vi "_Read RT Table.vi"(4 "error in (no error)":errorcluster, 6 "key":string, 7 "Simulator":bool) -> (0 "error out":errorcluster, 1 "Table":dbl[][](array[numeric]))   [LabVIEW 2015]
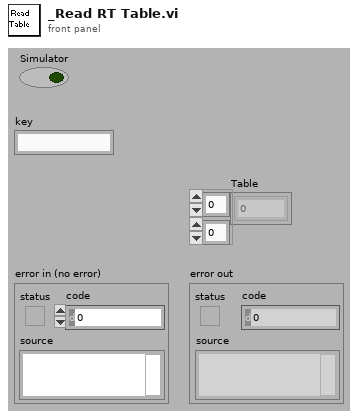
[diagram p1: front panel]
types:
  T1 = enum16{"open", "replace", "create", "open or create", "replace or create", "replace or create with confirmation"}
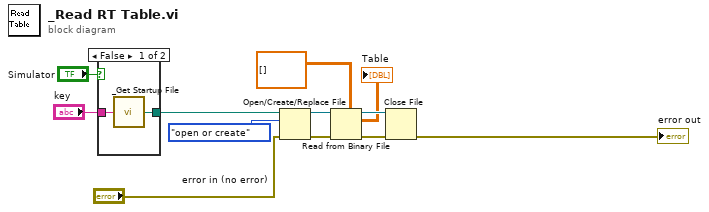
[diagram p0: block diagram]
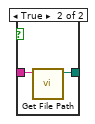
[diagram p2: hidden frame]
diagram:
  n1 = case shown="False" "Simulator" {
    tunnel: [w14 w15] -> w1
    tunnel: "key" -> [w13 w16]
    frame False {
      n2 = call "_Get Startup File.vi"("FileName"=w13) -> ("FilePath"=w14:path)
    }
    frame True {
      n3 = call "Get File Path.vi"("FileName"=w16) -> ("FilePath"=w15:path)  [unwired: 10 in]
    }
  }
  n4 = Open/Create/Replace File(file path (use dialog)=w1, error in="error in (no error)", operation (0:open)=T1."open or create") -> (refnum out=w2:refnum<file>, error out=w4:errorcluster)  [unwired: 3 in, 1 out]
  n5 = Read from Binary File(5:dbl[][] [], 8:w4, 11:w2) -> (0:w12:errorcluster, 2:→"Table":dbl[][], 3:w11:refnum<file>)  [unwired: 4 out]
  n6 = Close File(refnum=w11, error in=w12) -> (error out=→"error out":errorcluster)  [unwired: 1 out]
